vi "XNET Read (State FlexRay Comm).vi"(0 "session in":refnum<k21>, 11 "error in (no error)":errorcluster) -> (4 "session out":refnum<k21>, 6 "FlexRay comm":T1 {"fault code" format="%08x"; "FlexRay POC state" items=["Default Config"=0, "Ready"=1, "NormalActive"=2, "NormalPassive"=3, "Halt"=4, "Monitor"=5, "Config"=15]}, 15 "error out":errorcluster)   [LabVIEW 2018]
doc: "Reads the state of FlexRay communication using an XNET session."
uses:
  XNET FlexRay Comm.ctl
  XNET FlexRay POC State.ctl
  nixlvapi.dll
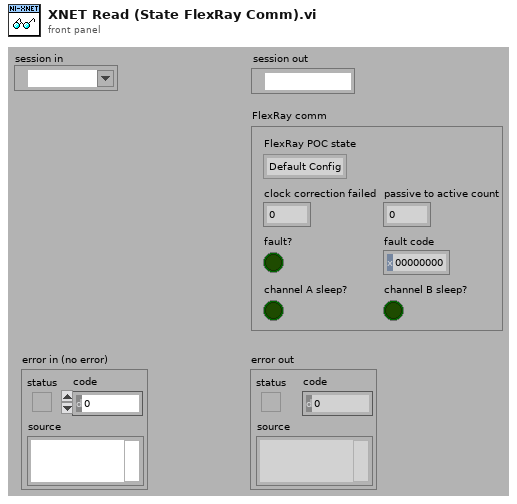
[diagram p1: front panel]
types:
  T1 = typedef "XNET FlexRay Comm.ctl" = cluster{"fault code":i32, "fault?":bool, "FlexRay POC state":T2, "clock correction failed":u8, "passive to active count":u8, "channel A sleep?":bool, "channel B sleep?":bool}
  T2 = typedef "XNET FlexRay POC State.ctl" = u8
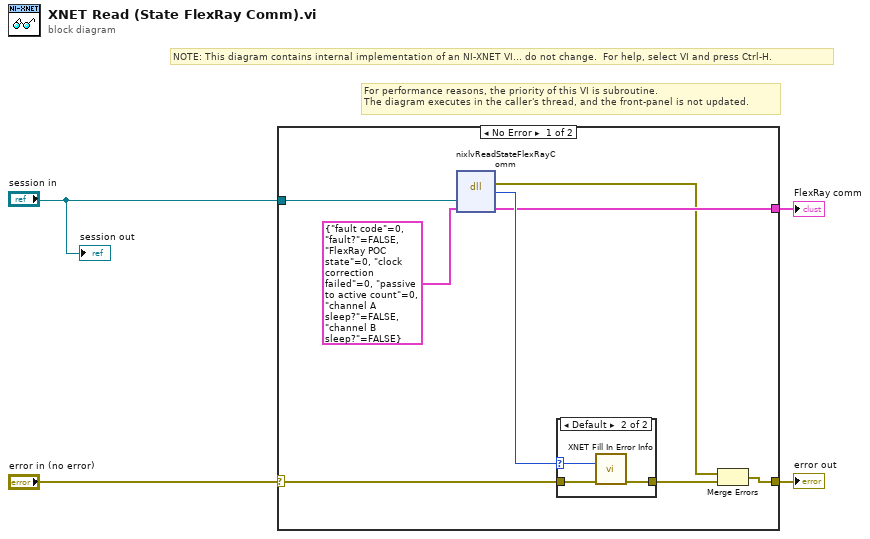
[diagram p0: block diagram]
diagram:
  # "For performance reasons, the priority of this VI is subroutine.\nThe diagram executes in the caller's thread, and the front-panel is not updated."
  # "NOTE: This diagram contains internal implementation of an NI-XNET VI... do not change.  For help, select VI and press Ctrl-H."
  n1 = case shown="No Error" "error in (no error)" {
    selector: "error in (no error)" -> [w11 w17]
    tunnel: "session in" -> [w12 _]
    tunnel: [w6 w17] -> w4
    tunnel: [w7 _] -> w1
    frame No Error {
      n2 = dll-call lib="nixlvapi.*" fn="nixlvReadStateFlexRayComm"("sessionRef"=w12, "flexRayComm"=T1 {"fault code"=0, "fault?"=FALSE, "FlexRay POC state"=0, "clock correction failed"=0, "passive to active count"=0, "channel A sleep?"=FALSE, "channel B sleep?"=FALSE} ("FlexRay comm")) -> (error out=w5:errorcluster, "return type"=w9:i32, "flexRayComm"=w7:T1)  [unwired: 3 in, 2 out]
      n3 = case shown="Default" w9 {
        selector: w9 -> [_ w14]
        tunnel: w11 -> [w13 w15]
        tunnel: [w13 w16] -> w10
        frame 0 {
        }
        frame Default {
          n4 = call "XNET Fill In Error Info.vi"("status code"=w14, "error in"=w15) -> ("error out"=w16:errorcluster)  [unwired: 13 out]
        }
      }
      n5 = Merge Errors(w5, w10) -> (w6:errorcluster)
    }
    frame Error {
    }
  }
  "error out" <- w4
  "FlexRay comm" <- w1
  "session out" <- "session in"
